vi "flames.vi"() -> ()   [LabVIEW 2018]
uses:
  <vilib>/Utility/error.llb/whitespace.ctl
  <vilib>/regexp/Match Regular Expression.xnode
panel:
  out "Result":string
  in  "Your Partner Name":string
  in  "Your Name":string
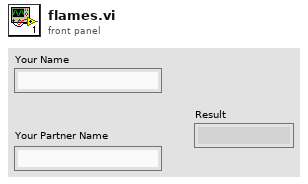
[diagram p1: front panel]
types:
  T1 = typedef "whitespace.ctl" = u16
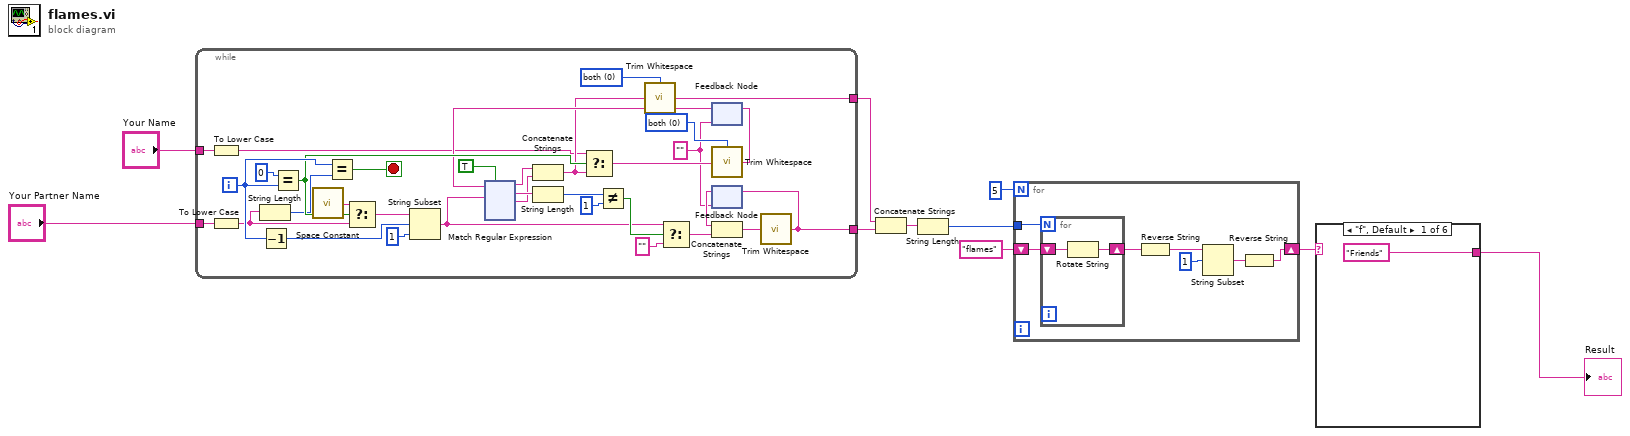
[diagram p0: block diagram]
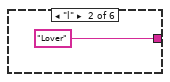
[diagram p2: hidden frame]
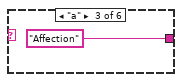
[diagram p3: hidden frame]
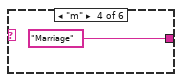
[diagram p4: hidden frame]
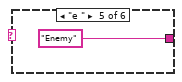
[diagram p5: hidden frame]
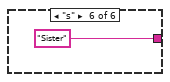
[diagram p6: hidden frame]
diagram:
  n1 = while {
    tunnel: "Your Name" -> [w14]
    tunnel: "Your Partner Name" -> [w11]
    tunnel: [w25] -> w4
    tunnel: [w15] -> w5
    i -> [w42]
    stop <- w41 stop-if-true
    w17 = "" ("trimmed string")
    w24 = T1 0 items=["both", "start of string", "end of string"] ("location (both)")
    w26 = T1 0 items=["both", "start of string", "end of string"] ("location (both)")
    n2 = To Lower Case(string=w14) -> (all lower case string=w13:string)
    n3 = To Lower Case(string=w11) -> (all lower case string=w12:string)
    n4 = String Length(string=w12) -> (length=w28:i32)
    n5 = Decrement(x=w42) -> (x-1=w29:i32)
    n6 = Equal?(x=0, y=w42) -> (x = y?=w32:bool)
    n7 = call <vilib>:"Space Constant.vi"() -> ("String"=w31:string)
    n8 = Equal?(x=w42, y=w28) -> (x = y?=w41:bool)
    n9 = Select(t=w31, s=w32, f=w12) -> (s? t:f=w33:string)
    n10 = String Subset(string=w33, offset (0)=w29, length (rest)=1 ("length (rest)")) -> (substring=w34:string)
    n11 = feedback #1(w17) -> (w21:string)
    n12 = xnode "Match Regular Expression"("input string"=w21, "regular expression"=w34, "ignore case? (F)"=TRUE) -> ("before match"=w40:string, "whole match"=w30:string, "after match"=w23:string)  [unwired: 3 in, 2 out]
    n13 = Concatenate Strings(w40, w23) -> (w20:string)
    n14 = String Length(string=w30) -> (length=w38:i32)
    n15 = Select(t=w13, s=w32, f=w20) -> (s? t:f=w27:string)
    n16 = Not Equal?(x=w38, y=1) -> (x != y?=w39:bool)
    n17 = call <vilib>:"Trim Whitespace.vi"("string"=w20, "location (both)"=w24) -> ("trimmed string"=w25:string)
    n18 = Select(t=w34, s=w39, f="") -> (s? t:f=w19:string)
    n19 = call <vilib>:"Trim Whitespace.vi"("string"=w27, "location (both)"=w26) -> ("trimmed string"=w22:string)
    n20 = feedback-in #1(w22) -> ()
    n21 = feedback #2(w17) -> (w18:string)
    n22 = Concatenate Strings(w18, w19) -> (w16:string)
    n23 = call <vilib>:"Trim Whitespace.vi"("string"=w16) -> ("trimmed string"=w15:string)  [unwired: 1 in]
    n24 = feedback-in #2(w15) -> ()
  }
  n25 = Concatenate Strings(w4, w5) -> (w3:string)
  n26 = String Length(string=w3) -> (length=w6:i32)
  n27 = for {
    N: 5 -> [_]
    shift-right: [w160] -> w2
    shift-left: "flames" ("String") -> [w165]
    tunnel: w6 -> [w159]
    n28 = for {
      N: w159 -> [_]
      shift-right: [w166] -> w164
      shift-left: w165 -> [w167]
      n29 = Rotate String(1:w167) -> (0:w166:string)
    }
    n30 = Reverse String(1:w164) -> (0:w162:string)
    n31 = String Subset(string=w162, offset (0)=1) -> (substring=w163:string)  [unwired: 1 in]
    n32 = Reverse String(1:w163) -> (0:w160:string)
  }
  n33 = case shown="\"f\", Default" w2 {
    tunnel: ["Friends" ("Output") "Lover" ("Output") "Affection" ("Output") "Marriage" "Enemy" "Sister"] -> w1
    frame "f", Default {
    }
    frame "l" {
    }
    frame "a" {
    }
    frame "m" {
    }
    frame "e " {
    }
    frame "s" {
    }
  }
  "Result" <- w1
